vi "Configure Smoothing.vi"(8 "error in (no error)":errorcluster, 9 "Response Speed (0: Slow)":i32(ring) items=["Slow", "Medium", "Fast"], 10 "Enable Smoothing (F: Disable)":bool, 11 "VISA resource name":refnum<visa-resource-name>) -> (0 "error out":errorcluster, 3 "VISA resource name out":refnum<visa-resource-name>)   [LabVIEW 2020, in "Agilent 3446X Series.lvlib"]
doc: "Enables or disables statistics computation.\n\n<b>Note(s):</b>\nThis vi is not supported for EDU34450A model."
uses:
  Agilent 3446X Series.lvlib
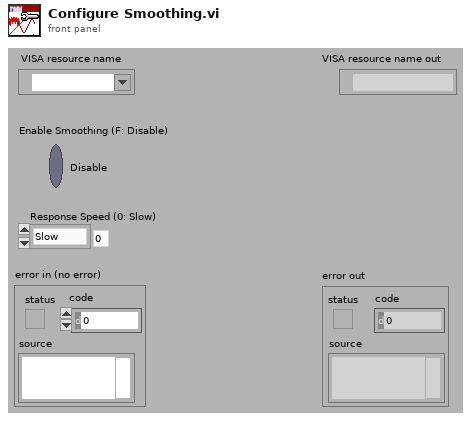
[diagram p1: front panel]
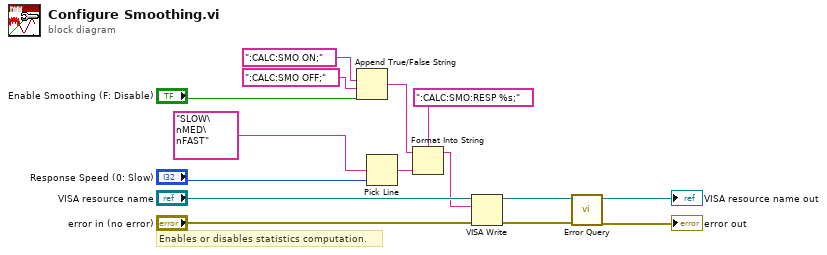
[diagram p0: block diagram]
diagram:
  # "Enables or disables statistics computation."
  n1 = Append True/False String(1:"Enable Smoothing (F: Disable)", 2:":CALC:SMO OFF;", 3:":CALC:SMO ON;") -> (0:w6:string)  [unwired: 1 out]
  n2 = Pick Line(multi-line string="SLOW\nMED\nFAST", line index="Response Speed (0: Slow)") -> (output string=w2:string)  [unwired: 1 in]
  n3 = Format Into String(format string=":CALC:SMO:RESP %s;", initial string=w6, w2) -> (resulting string=w5:string)  [unwired: 1 in, 1 out]
  n4 = VISA Write(VISA resource name="VISA resource name", write buffer=w5, error in (no error)="error in (no error)") -> (VISA resource name out=w11:refnum<visa-resource-name>, error out=w10:errorcluster)  [unwired: 1 out]
  n5 = call "Error Query.vi"("error in (no error)"=w10, "VISA resource name"=w11) -> ("error out"=→"error out":errorcluster, "VISA resource name out"=→"VISA resource name out":refnum<visa-resource-name>)  [unwired: 8 out]
